vi "BotSpeak_VariableFinder.vi"(2 "Reset?":bool, 3 "Var #?":bool, 4 "variable name":string) -> (0 "codes":u8[](array[numeric]), 1 "Variables":string[](array[string]))   [LabVIEW 2014]
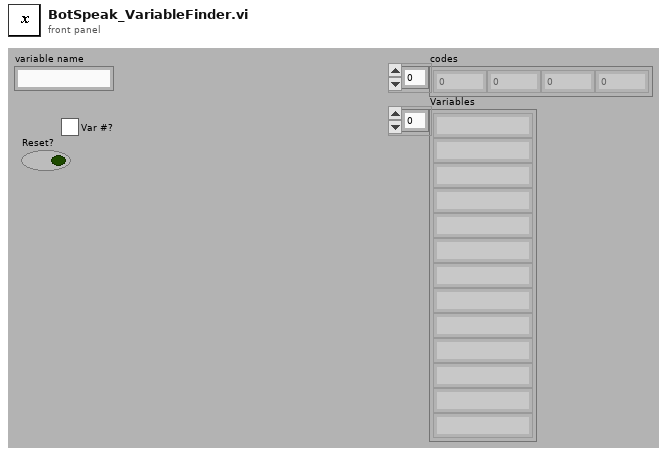
[diagram p1: front panel]
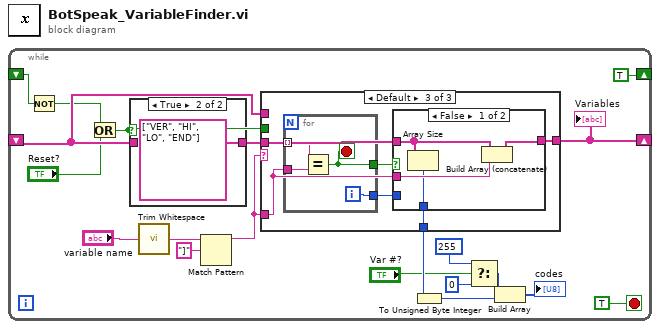
[diagram p0: block diagram]
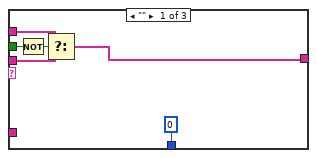
[diagram p2: hidden frame]
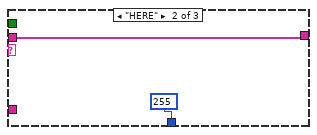
[diagram p3: hidden frame]
diagram:
  n1 = while {
    shift-right: [w11] -> _
    shift-left: _ -> [w10]
    shift-right: [TRUE] -> _
    shift-left: _ -> [w4]
    stop <- TRUE stop-if-true
    n2 = Not(x=w4) -> (.not. x?=w3:bool)
    n3 = Or(x=w3, y="Reset?") -> (x .or. y?=w1:bool)
    n4 = case shown="True" w1 {
      tunnel: [w45 string[] ["VER", "HI", "LO", "END"] ("Variables")] -> w20
      tunnel: w10 -> [w45 _]
      frame False {
      }
      frame True {
      }
    }
    n5 = call <vilib>:"Trim Whitespace.vi"("string"="variable name") -> ("trimmed string"=w6:string)  [unwired: 1 in]
    n6 = Match Pattern(string=w6, regular expression="]") -> (before substring=w7:string)  [unwired: 1 in, 3 out]
    n7 = case shown="Default" w7 {
      tunnel: w20 -> [w22 w27 w33]
      tunnel: w7 -> [_ _ w32]
      tunnel: [0 255 w30] -> w15
      tunnel: [w21 w27 w29] -> w11
      tunnel: w10 -> [w23 _ _]
      tunnel: w1 -> [w25 _ _]
      frame "" {
        n8 = Not(x=w25) -> (.not. x?=w24:bool)
        n9 = Select(t=w23, s=w24, f=w22) -> (s? t:f=w21:string[])
      }
      frame "HERE" {
      }
      frame Default {
        n10 = for {
          tunnel: w33 -> [w42] mode=indexing
          tunnel: w32 -> [w43]
          tunnel: [w44] -> w34
          tunnel: [w41] -> w31
          i -> [w41]
          stop <- w44 stop-if-true
          n11 = Equal?(x=w42, y=w43) -> (x = y?=w44:bool)
        }
        n12 = case shown="False" w34 {
          tunnel: w32 -> [w37 _]
          tunnel: w33 -> [w36 w40]
          tunnel: [w38 w40] -> w29
          tunnel: [w35 w39] -> w30
          tunnel: w31 -> [_ w39]
          frame False {
            n13 = Array Size(array=w36) -> (size(s)=w35:i32)
            n14 = Build Array (concatenate)(w36, w37) -> (w38:string[])
          }
          frame True {
          }
        }
      }
    }
    "Variables" <- w11
    n15 = To Unsigned Byte Integer(number=w15) -> (unsigned 8bit integer=w17:u8)
    n16 = Select(t=u8 255 ("element"), s="Var #?", f=u8 0 ("element")) -> (s? t:f=w19:u8)
    n17 = Build Array(w19, w17) -> (→"codes":u8[])
  }
